vi "Rename Object Labels.vi"(6 "Post":string, 8 "error in":errorcluster, 9 "Pre":string, 10 "Class Ref":refnum<vi>) -> (0 "error out":errorcluster)   [LabVIEW 2020, in "_Rename.lvlib" / "_Rename.lvclass"]
uses:
  _Rename.lvclass
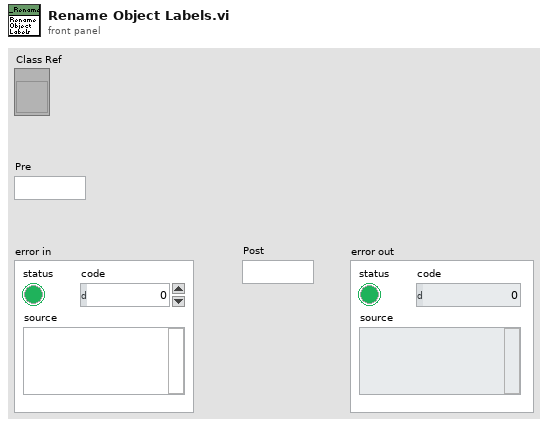
[diagram p1: front panel]
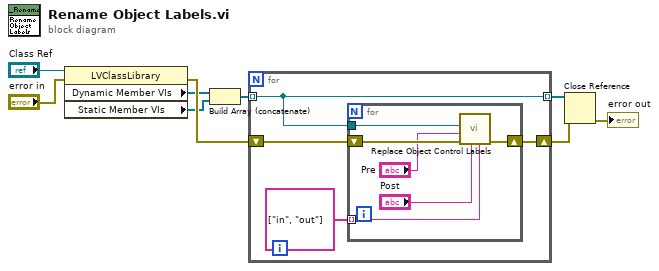
[diagram p0: block diagram]
diagram:
  n1 = property class="LVClassLibrary"(reference="Class Ref", error in="error in") -> (error out=w9:errorcluster, "Dynamic Member VIs"=w6:refnum<vi>[], "Static Member VIs"=w7:refnum<vi>[])  [unwired: 1 out]
  n2 = Build Array (concatenate)(w6, w7) -> (w8:refnum<vi>[])
  n3 = for {
    tunnel: w8 -> [w11] mode=indexing
    shift-right: [w10] -> w4
    shift-left: w9 -> [w13]
    tunnel: [w11] -> w5 mode=indexing
    n4 = for {
      tunnel: w11 -> [w14]
      tunnel: string[] ["in", "out"] -> [w18] mode=indexing
      shift-right: [w17] -> w10
      shift-left: w13 -> [w19]
      n5 = call "Replace Object Control Labels.vi"("in / out"=w18, "Post"="Post", "error in"=w19, "Pre"="Pre", "VI Ref"=w14) -> ("error out"=w17:errorcluster)  [unwired: 6 in]
    }
  }
  n6 = Close Reference(reference=w5, error in (no error)=w4) -> (error out=→"error out":errorcluster)
